vi "readFromXML.vi"(8 "error in (no error)":errorcluster, 10 "XML in":string, 11 "SetEngineerAccessMode in":refnum<class "SetEngineerAccessMode.lvclass">) -> (0 "error out":errorcluster, 3 "SetEngineerAccessMode out":refnum<class "SetEngineerAccessMode.lvclass">)   [LabVIEW 2014, in "TCSDataDefinitions.lvlib" / "TCSCommand.lvlib" / "SetAccessMode.lvlib" / "SetEngineerAccessMode.lvclass"]
uses:
  SetEngineerAccessMode.lvclass
  SetEngineerAccessMode.lvclass/SetEngineerAccessMode.ctl
  SetAccessMode/SetAccessMode.lvclass
  <userlib>/Common/XML/XMLParser/XMLParser.lvclass
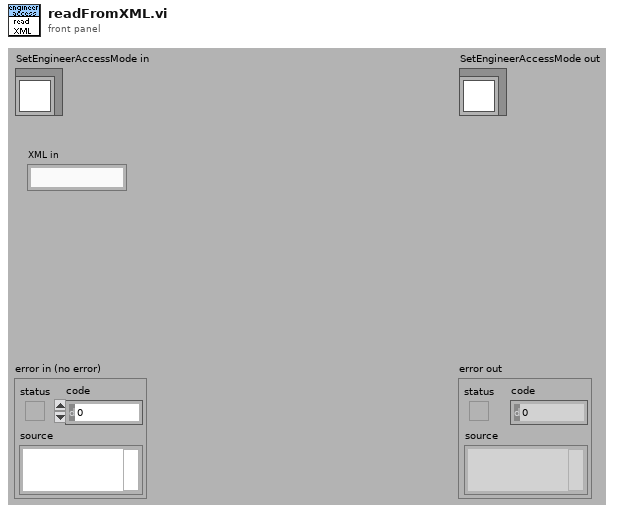
[diagram p1: front panel]
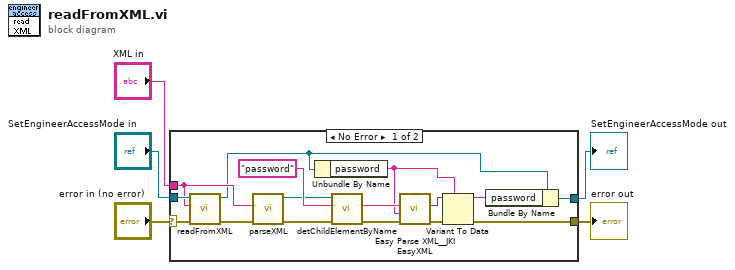
[diagram p0: block diagram]
diagram:
  n1 = case shown="No Error" "error in (no error)" {
    selector: "error in (no error)" -> [w16 w23]
    tunnel: [w9 w23] -> w4
    tunnel: [w14 w22] -> w2
    tunnel: "SetEngineerAccessMode in" -> [w21 w22]
    tunnel: "XML in" -> [w19 _]
    frame No Error {
      n2 = call-parent "readFromXML.vi"("error in (no error)"=w16, "XML in"=w19, "SetAccessMode in"=w21) -> ("error out"=w20:errorcluster, "SetAccessMode out"=w15:refnum<class "SetEngineerAccessMode.lvclass">)  [unwired: 7 out]
      n3 = call <userlib>:"parseXML.vi"("error in (no error)"=w20, "XMLString in"=w19) -> ("error out"=w17:errorcluster, "Element out"=w6:refnum<class "XMLParser.lvclass">)  [unwired: 8 in]
      n4 = Unbundle By Name(w15) -> ("password"=w8:string)
      n5 = call <userlib>:"detChildElementByName.vi"("error in (no error)"=w17, "childName"="password" ("ChildName"), "Element in"=w6) -> ("error out"=w10:errorcluster, "childXML"=w11:string)  [unwired: 5 in, 2 out]
      n6 = call <vilib>:"Easy Parse XML__JKI EasyXML.vi"("error in (no error)"=w10, "LabVIEW Data (Type)"=w8, "XML String"=w11) -> ("error out"=w13:errorcluster, "LabVIEW Data"=w12:variant)  [unwired: 7 in]
      n7 = Variant To Data(error in=w13, type=w8, Variant=w12) -> (data=w7:string, error out=w9:errorcluster)
      n8 = Bundle By Name(cluster=w15, "password"=w7) -> (w14:refnum<class "SetEngineerAccessMode.lvclass">)
    }
    frame Error {
    }
  }
  "error out" <- w4
  "SetEngineerAccessMode out" <- w2
